vi "Show Splitter Settings UI.vi"(8 "Error In":errorcluster, 10 "Splitter":refnum<class "Splitter.lvclass">, 11 "Splitter Settings UI in":refnum<class "Splitter Settings UI.lvclass">) -> (0 "Error Out":errorcluster, 3 "Splitter Settings UI out":refnum<class "Splitter Settings UI.lvclass">)   [LabVIEW 2015, in "Splitter Settings UI.lvlib" / "Splitter Settings UI.lvclass"]
uses:
  Splitter Settings UI.lvclass
  Classes/Splitter/Splitter.lvclass
  <vilib>/ActorFramework/Actor/Actor.lvclass/Actor.ctl
  <vilib>/ActorFramework/Message Enqueuer/Message Enqueuer.lvclass/Message Enqueuer.ctl
  Splitter Settings UI.lvclass/Splitter Settings UI.ctl
  <vilib>/ActorFramework/Message Enqueuer/Init from Existing Queue.vi
  <vilib>/ActorFramework/Message Enqueuer/Message Enqueuer.lvclass
  <vilib>/MGI/Panel Manager/Panel Actor/Panel Actor Messages/Show Panel Msg/Show Panel Msg.lvclass
  <vilib>/ActorFramework/Actor/Actor.lvclass
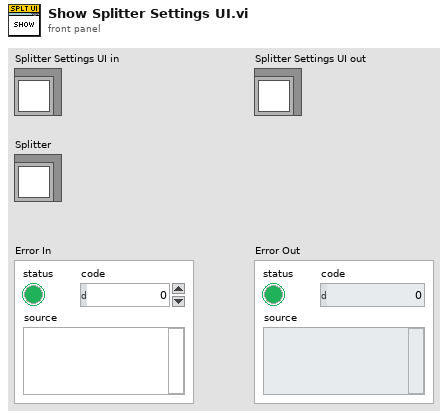
[diagram p1: front panel]
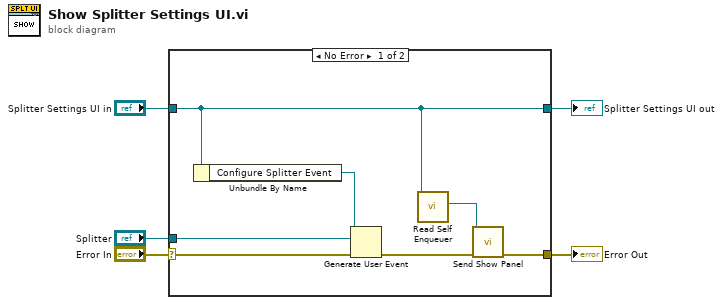
[diagram p0: block diagram]
diagram:
  n1 = case shown="No Error" "Error In" {
    selector: "Error In" -> [w12 w14]
    tunnel: [w7 w14] -> w2
    tunnel: [w9 w13] -> w4
    tunnel: "Splitter Settings UI in" -> [w9 w13]
    tunnel: "Splitter" -> [w10 _]
    frame No Error {
      n2 = Unbundle By Name(w9) -> ("Configure Splitter Event"=w11:refnum<user-event>)
      n3 = Generate User Event(user event=w11, event data cluster=w10, error in=w12) -> (error out=w8:errorcluster)  [unwired: 1 in, 1 out]
      n4 = call <vilib>:"Read Self Enqueuer.vi"("Actor"=w9) -> ("Self Enqueuer"=w6:refnum<class "Message Enqueuer.lvclass">)  [unwired: 10 in]
      n5 = call <vilib>:"Send Show Panel.vi"("Error In"=w8, "Message Enqueuer in"=w6) -> ("Error Out"=w7:errorcluster)  [unwired: 8 in, 1 out]
    }
    frame Error {
    }
  }
  "Splitter Settings UI out" <- w4
  "Error Out" <- w2
